vi "ZMQ.TestLauncher.REP.vi"() -> ()   [LabVIEW 2020, in "RemoteControl.ZMQ.lvclass"]
uses:
  RemoteControl.ZMQ.lvclass
  <vilib>/JKI/JKI SMO/SMO/SMO.lvclass
  <vilib>/JKI/JKI SMO/SMO/Typedefs/SMOState --Enum.ctl
  <vilib>/addons/zeromq/socket_type.ctl
  <vilib>/addons/zeromq/zeromq.lvlib
  Typedefs/ZMQ Config.ctl
  C:/Program Files (x86)/National Instruments/LabVIEW 2020/vi.lib/JKI/JKI SMO/SMO/SMO.lvclass
  <vilib>/addons/zeromq/zmq_socket.lvclass
  Typedefs/PublicEvents--ZMQ.receiveMessage.ctl
panel:
  in  "reply message":string[](array[string])
  out "message":T1
  out "SMO State":T2
  out "error out":errorcluster
  in  "Stop":bool
  # "REP SMO Test Launcher"
  # "For instructions on how to use the JKI State Machine Objects, examples and video tutorials, visit:\nhttp://jki.net/state-machine-objects/\n\nJKI State Machine Objects™\nhttp://jki.net/state-machine-objects/\nCopyright (C) 2005-2015, JKI <info@jki.net>\nALL RIGHTS RESERVED"
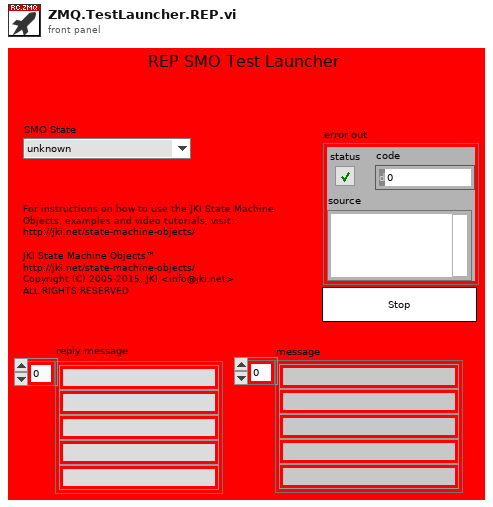
[diagram p1: front panel]
types:
  T1 = typedef "RemoteControl.ZMQ.lvclass/PublicEvents--ZMQ.receiveMessage.ctl" = string[]
  T2 = typedef "SMO.lvclass/SMOState --Enum.ctl" = enum16{"unknown", "Created", "Started", "Stopped"}
  T3 = typedef "RemoteControl.ZMQ.lvclass/ZMQ Config.ctl" = cluster{"Socket":refnum<class "zmq_socket.lvclass">, "socket type":T4, "endpoint":string, "filter":string}
  T4 = typedef "zeromq.lvlib/socket_type.ctl" = enum8{"ZMQ_PAIR", "ZMQ_PUB", "ZMQ_SUB", "ZMQ_REQ", "ZMQ_REP", "ZMQ_DEALER", "ZMQ_ROUTER", "ZMQ_PULL", "ZMQ_PUSH", "ZMQ_XPUB", "ZMQ_XSUB"}
  T5 = typedef "SMO.lvclass/Public Events.ctl" = cluster{"Error":refnum<user-event>, "State":refnum<user-event>, "Reserve State":refnum<user-event>}
  T6 = typedef "RemoteControl.ZMQ.lvclass/PublicEvents--Cluster.ctl" = cluster{"receiveMessage":refnum<user-event>}
  T7 = cluster{"Event Registration Refnum":refnum<event-registration>}
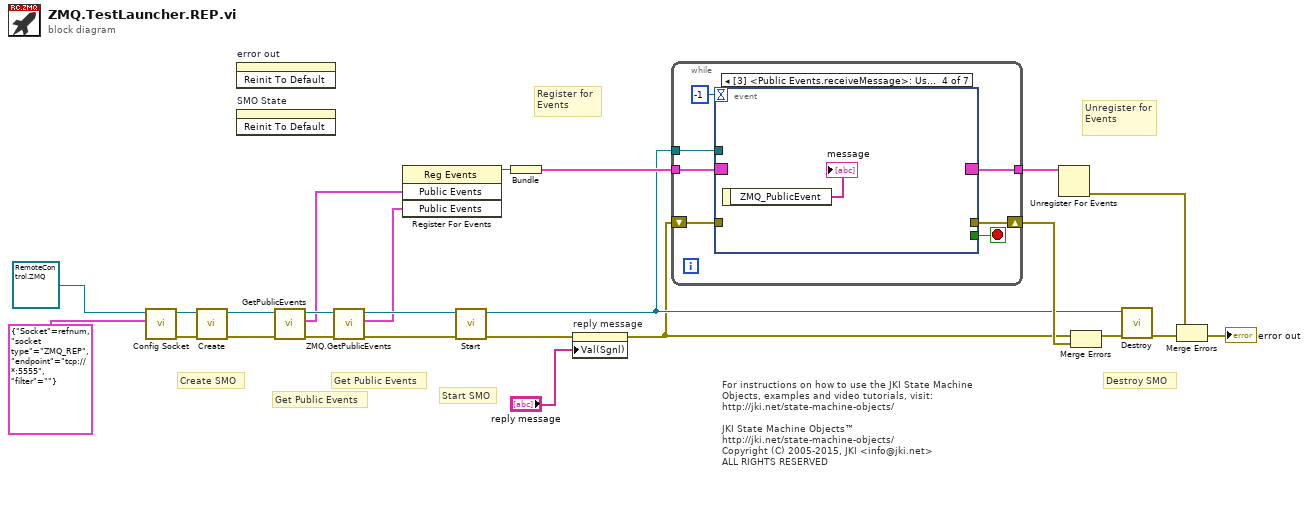
[diagram p0: block diagram]
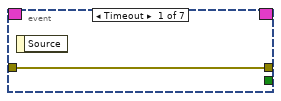
[diagram p2: hidden frame]
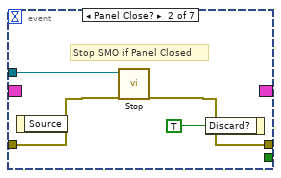
[diagram p3: hidden frame]
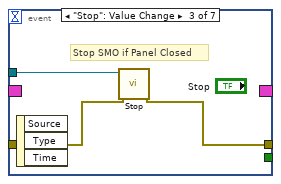
[diagram p4: hidden frame]
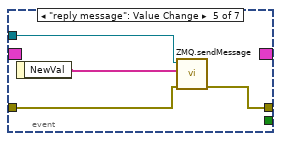
[diagram p5: hidden frame]
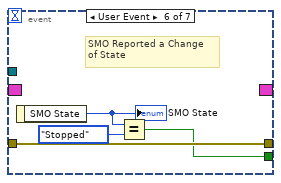
[diagram p6: hidden frame]
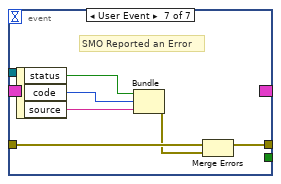
[diagram p7: hidden frame]
diagram:
  # "Get Public Events"
  # "For instructions on how to use the JKI State Machine Objects, examples and video tutorials, visit:\nhttp://jki.net/state-machine-objects/\n\nJKI State Machine Objects™\nhttp://jki.net/state-machine-objects/\nCopyright (C) 2005-2015, JKI <info@jki.net>\nALL RIGHTS RESERVED"
  # "Get Public Events"
  # "Start SMO"
  # "Destroy SMO"
  # "Create SMO"
  # "Unregister for Events"
  # "Register for Events"
  n1 = call "Config Socket.vi"("Socket Config"=T3 {"Socket"=refnum, "socket type"=enum."ZMQ_REP", "endpoint"="tcp://*:5555", "filter"=""}, "ZMQ in"=refnum<class "RemoteControl.ZMQ.lvclass"> refnum ("SMO.Template.lvclass")) -> ("error out"=w10:errorcluster, "ZMQ out"=w11:refnum<class "RemoteControl.ZMQ.lvclass">)  [unwired: 8 in]
  n2 = call <vilib>:"Create.vi"("error in (no error)"=w10, "SMO"=w11) -> ("error out"=w16:errorcluster, "SMO out"=w17:refnum<class "RemoteControl.ZMQ.lvclass">)  [unwired: 7 in, 1 out]
  n3 = invoke on="error out" class="Clust (strict)" method="Reinit To Default"() -> ()  [unwired: 3 in, 3 out]
  n4 = invoke on="SMO State" class="Enum (strict)" method="Reinit To Default"() -> ()  [unwired: 3 in, 3 out]
  n5 = call <vilib>:"GetPublicEvents.vi"("error in (no error)"=w16, "SMO"=w17) -> ("error out"=w7:errorcluster, "Public Events"=w5:T5, "SMO out"=w8:refnum<class "RemoteControl.ZMQ.lvclass">)  [unwired: 7 in]
  n6 = call "ZMQ.GetPublicEvents.vi"("error in (no error)"=w7, "ZMQ"=w8) -> ("error out"=w14:errorcluster, "Public Events"=w6:T6, "ZMQ out"=w15:refnum<class "RemoteControl.ZMQ.lvclass">)  [unwired: 7 in]
  n7 = register-events(w5, w6) -> (reference out=w9:refnum<event-registration>)  [unwired: 2 in, 1 out]
  n8 = call <vilib>:"Start.vi"("error in (no error)"=w14, "SMO"=w15) -> ("error out"=w3:errorcluster, "SMO out"=w13:refnum<class "RemoteControl.ZMQ.lvclass">)  [unwired: 8 in]
  n9 = Bundle("Event Registration Refnum"=w9) -> (w23:T7)  [unwired: 1 in]
  n10 = property on="reply message" class="Arr (strict)"(error in=w3, "Val(Sgnl)"="reply message") -> (error out=w2:errorcluster)  [unwired: 1 in, 1 out]
  n11 = while {
    shift-right: [w30] -> w22
    shift-left: w2 -> [w25]
    tunnel: w23 -> [w29]
    tunnel: [w28] -> w24
    tunnel: w13 -> [w27]
    stop <- w31 stop-if-true
    n12 = event shown="[3] <Public Events.receiveMessage>: User Event" {
      selector: w29 -> [_ _ _ _ _ _ _]
      dyn-events: [_ _ _ _ _ _ _] -> w28
      timeout: -1 -> [_ _ _ _ _ _ _]
      tunnel: [_ _ _ _ _ w45 _] -> w31
      tunnel: w27 -> [_ w36 w39 _ w43 _ _]
      tunnel: [w32 w35 w38 _ w44 w48 w52] -> w30
      tunnel: w25 -> [w32 w34 w37 _ w42 w48 w50]
      event Timeout {
        n13 = event-data() -> ()  [unwired: 1 in, 1 out]
      }
      event Panel Close? {
        # "Stop SMO if Panel Closed"
        n14 = event-data() -> ()  [unwired: 1 in, 1 out]
        n15 = call <vilib>:"Stop.vi"("error in (no error)"=w34, "SMO"=w36) -> ("error out"=w35:errorcluster)  [unwired: 8 in, 1 out]
        n16 = event-data("Discard?"=TRUE ("OK")) -> ()  [unwired: 1 in, 1 out]
      }
      event "Stop": Value Change {
        # "Stop SMO if Panel Closed"
        n17 = event-data() -> ()  [unwired: 1 in, 3 out]
        n18 = call <vilib>:"Stop.vi"("error in (no error)"=w37, "SMO"=w39) -> ("error out"=w38:errorcluster)  [unwired: 8 in, 1 out]
      }
      event User Event {
        n19 = event-data() -> ("ZMQ_PublicEvent"=→"message":T1)  [unwired: 1 in]
      }
      event "reply message": Value Change {
        n20 = event-data() -> ("NewVal"=w41:string[])  [unwired: 1 in]
        n21 = call "ZMQ.sendMessage.vi"("error in (no error)"=w42, "message"=w41, "ZMQ"=w43) -> ("error out"=w44:errorcluster)  [unwired: 7 in, 1 out]
      }
      event User Event {
        # "SMO Reported a Change\nof State"
        n22 = event-data() -> ("SMO State"=w47:T2)  [unwired: 1 in]
        "SMO State" <- w47
        n23 = Equal?(x=w47, y=SMOState_--Enum."Stopped") -> (x = y?=w45:bool)
      }
      event User Event {
        # "SMO Reported an Error"
        n24 = event-data() -> ("status"=w51:bool, "code"=w54:i32, "source"=w53:string)  [unwired: 1 in]
        n25 = Bundle("status"=w51, "code"=w54, "source"=w53) -> (w49:errorcluster)  [unwired: 1 in]
        n26 = Merge Errors(w50, w49) -> (w52:errorcluster)
      }
    }
  }
  n27 = Unregister For Events(event registration refnum=w24) -> (error out=w21:errorcluster)  [unwired: 1 in]
  n28 = Merge Errors(w2, w22) -> (w18:errorcluster)
  n29 = call <vilib>:"Destroy.vi"("error in (no error)"=w18, "SMO"=w13) -> ("error out"=w19:errorcluster)  [unwired: 9 in]
  n30 = Merge Errors(w21, w19) -> (→"error out":errorcluster)
